vi "instance count allowed.vi"(8 "error in":errorcluster, 11 "Tagbus PID Module configuration in":refnum<class "PID Module configuration.lvclass">) -> (0 "error out":errorcluster, 2 "instances allowed":i32, 3 "Tagbus PID Module configuration out":refnum<class "PID Module configuration.lvclass">)   [LabVIEW 2014, in "PID Module configuration.lvclass"]
uses:
  PID Module configuration.lvclass
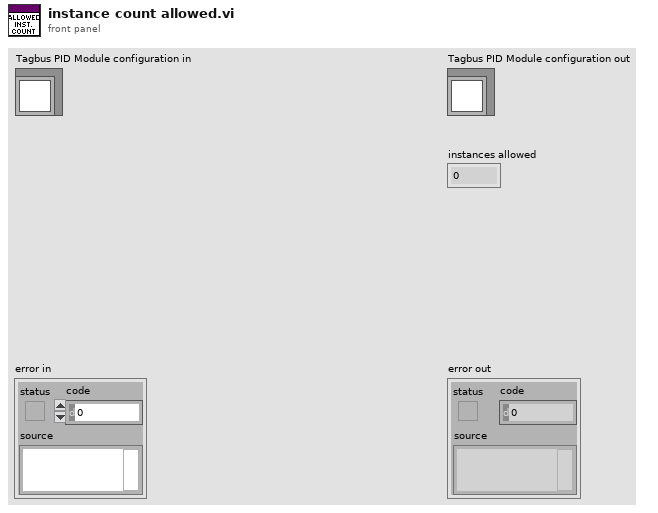
[diagram p1: front panel]
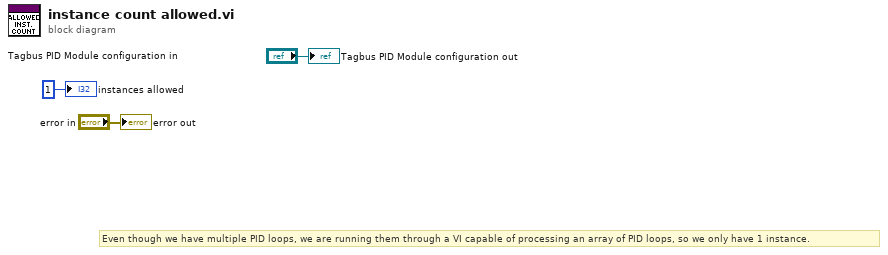
[diagram p0: block diagram]
diagram:
  # "Even though we have multiple PID loops, we are running them through a VI capable of processing an array of PID loops, so we only have 1 instance."
  "error out" <- "error in"
  "Tagbus PID Module configuration out" <- "Tagbus PID Module configuration in"
  "instances allowed" <- 1 ("instances allowed")
